vi "Vision Align.vi"(0 "Z Drive PID Gains":T4, 1 "output range":cluster{"output high":dbl, "output low":dbl}, 5 "Needed Angle":dbl, 7 "Current Angle":dbl, 9 "GyroDevRef":T1={"DevStatus"={"status"=FALSE, "code"=0, "source"=""}, "Analog Channel"=enum."AI 1", "Offset"=0.0, "Gain (VoltsPerDegree/Second)"=0.0, "Gyro Type"=enum."Analog", "Handle"=0, "SPI Bus"=enum."Invalid", "Device Found"=FALSE, "Sample Rate"=1.0, "Calibrate On Open"=FALSE} {"Sample Rate" min=0.25 max=100.0 step=0.25}, 11 "error in":errorcluster) -> (15 "Error Out":errorcluster)   [LabVIEW 2016]
uses:
  <vilib>/Rock Robotics/WPI/Gyro/WPI_GyroDevRef.ctl
  <vilib>/Rock Robotics/SystemInterfaces/AI/FPGA_AIChannel.ctl
  <vilib>/Rock Robotics/SystemInterfaces/spilib/spi_bus.ctl
  <vilib>/addons/control/pid/pid.llb/PID (DBL).vi
  <vilib>/addons/control/pid/NI_PID_pid.lvlib
panel:
  # "Analog"
  # "XRS"
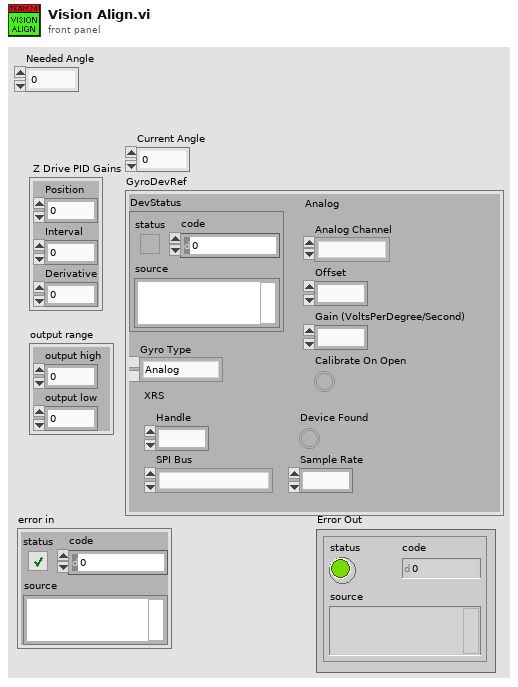
[diagram p1: front panel]
types:
  T1 = typedef "WPI_GyroDevRef.ctl" = cluster{"DevStatus":errorcluster, "Analog Channel":T2, "Offset":dbl, "Gain (VoltsPerDegree/Second)":dbl, "Gyro Type":enum16{"Analog", "XRS450"}, "Handle":i32, "SPI Bus":T3, "Device Found":bool, "Sample Rate":dbl, "Calibrate On Open":bool}
  T2 = typedef "FPGA_AIChannel.ctl" = enum8{"AI 0", "AI 1", "AI 2", "AI 3", "AI MXP 0", "AI MXP 1", "AI MXP 2", "AI MXP 3", "Invalid"}
  T3 = typedef "spi_bus.ctl" = enum16{"SPI On-Board, CS0", "SPI On-Board, CS1", "SPI On-Board, CS2", "SPI On-Board, CS3", "SPI MXP", "Invalid"}
  T4 = cluster{"Position":dbl, "Interval":dbl, "Derivative":dbl}
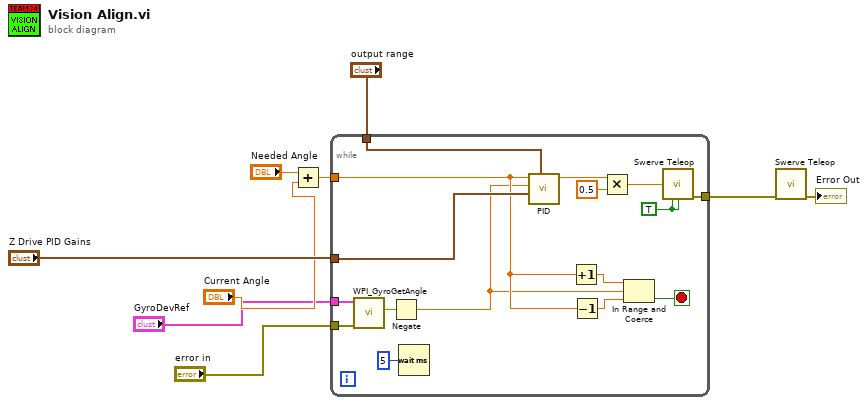
[diagram p0: block diagram]
diagram:
  n1 = Add(x="Needed Angle", y="Current Angle") -> (x+y=w5:dbl)
  n2 = while {
    tunnel: w5 -> [w14]
    tunnel: "Z Drive PID Gains" -> [w21]
    tunnel: "output range" -> [w25]
    tunnel: [w19] -> w8
    tunnel: "GyroDevRef" -> [w13]
    tunnel: "error in" -> [w12]
    stop <- w24 stop-if-true
    w18 = TRUE ("Robot Centric?")
    n3 = call <vilib>:"WPI_GyroGetAngle.vi"("error in"=w12, "GyroDevRef"=w13) -> ("Angle"=w11:dbl)  [unwired: 5 in, 4 out]
    n4 = Negate(x=w11) -> (-x=w10:dbl)
    n5 = Wait (ms)(milliseconds to wait=u32 5) -> ()  [unwired: 1 out]
    n6 = call-poly <vilib>:"PID.vi"("output range"=w25, "PID gains"=w21, "process variable"=w10, "setpoint"=w14) -> ("output"=w23:dbl)  [unwired: 6 in, 1 out]
    n7 = Increment(x=w14) -> (x+1=w17:dbl)
    n8 = Decrement(x=w14) -> (x-1=w16:dbl)
    n9 = Multiply(x=w23, y=0.5) -> (x*y=w20:dbl)
    n10 = In Range and Coerce(upper limit=w17, x=w10, lower limit=w16) -> (In Range?=w24:bool)  [unwired: 1 out]
    n11 = call "Swerve Teleop.vi"("Z"=w20, "Robot Centric?"=w18, "Autonomous?"=w18) -> ("Error Out"=w19:errorcluster)  [unwired: 8 in, 4 out]
  }
  n12 = call "Swerve Teleop.vi"("Error In"=w8) -> ("Error Out"=→"Error Out":errorcluster)  [unwired: 10 in, 4 out]
